vi "Read cfg file folder.vi"(8 "error in (no error)":errorcluster, 11 "[V] Sys Cfg Base in":refnum<class "[V] Sys Cfg Base.lvclass">) -> (0 "error out":errorcluster, 2 "cfg file folder":path, 3 "[V] Sys Cfg Base out":refnum<class "[V] Sys Cfg Base.lvclass">)   [LabVIEW 2023, in "[V] Sys Cfg Base.lvlib" / "[V] Sys Cfg Base.lvclass"]
uses:
  [V] Sys Cfg Base.lvclass
  [V] Sys Cfg Base.lvclass/[V] Sys Cfg Base.ctl
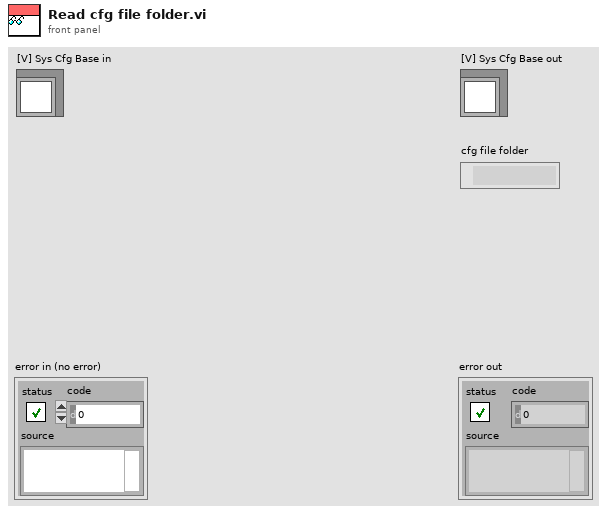
[diagram p1: front panel]
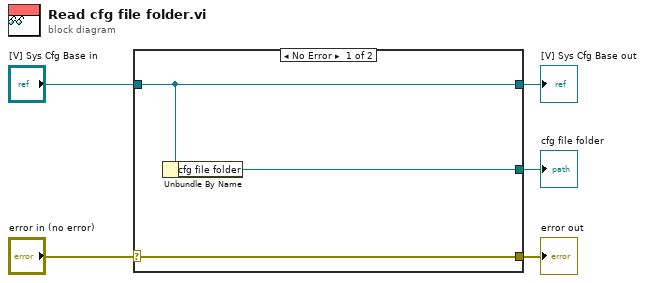
[diagram p0: block diagram]
diagram:
  n1 = case shown="No Error" "error in (no error)" {
    selector: "error in (no error)" -> [w8 w9]
    tunnel: [w8 w9] -> w4
    tunnel: [w7 w10] -> w2
    tunnel: "[V] Sys Cfg Base in" -> [w7 w10]
    tunnel: [w6 _] -> w1
    frame No Error {
      n2 = Unbundle By Name(w7) -> ("cfg file folder"=w6:path)
    }
    frame Error {
    }
  }
  "error out" <- w4
  "[V] Sys Cfg Base out" <- w2
  "cfg file folder" <- w1
